vi "写入控件ID.vi"(8 "error in (no error)":errorcluster caption="错误输入（无错误）", 10 "控件ID":u32, 11 "程序输入":refnum<class "程序.lvclass">) -> (0 "error out":errorcluster caption="错误输出", 3 "程序输出":refnum<class "程序.lvclass">)   [LabVIEW 2018, in "程序.lvclass"]
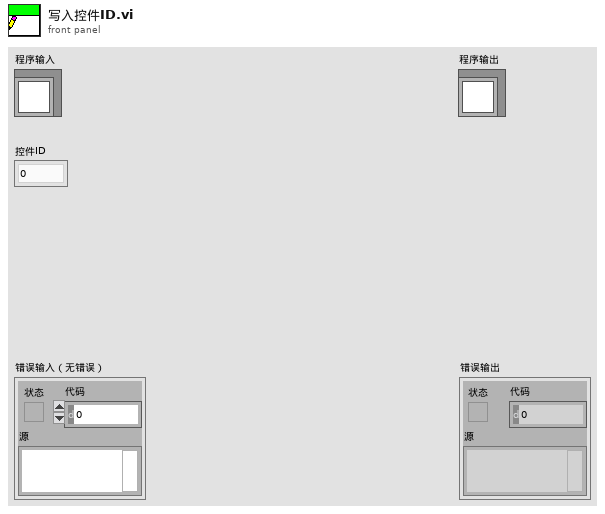
[diagram p1: front panel]
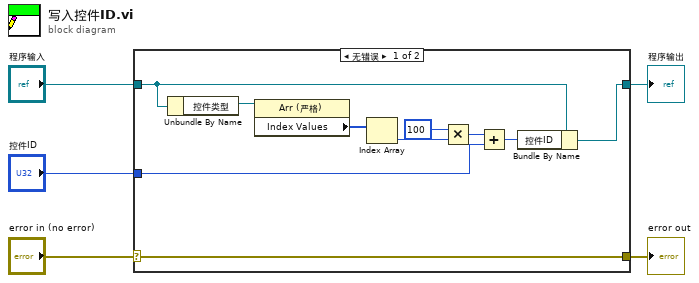
[diagram p0: block diagram]
diagram:
  n1 = case shown="无错误" "error in (no error)" {
    selector: "error in (no error)" -> [w15 w16]
    tunnel: [w15 w16] -> w4
    tunnel: [w14 w17] -> w2
    tunnel: "程序输入" -> [w13 w17]
    tunnel: "控件ID" -> [w7 _]
    frame No Error {
      n2 = Unbundle By Name(w13) -> ("控件类型"=w12:refnum<vi>)
      n3 = property class="Arr (严格)"(reference=w12) -> ("Index Values"=w11:u32[])  [unwired: 1 in, 2 out]
      n4 = Index Array(array=w11) -> (element=w10:u32)  [unwired: 1 in]
      n5 = Multiply(x=u32 100, y=w10) -> (x*y=w8:u32)
      n6 = Add(x=w8, y=w7) -> (x+y=w6:u32)
      n7 = Bundle By Name(cluster=w13, "控件ID"=w6) -> (w14:refnum<class "程序.lvclass">)
    }
    frame Error {
    }
  }
  "error out" <- w4
  "程序输出" <- w2
